vi "Equal.vi"(0 "VI Reference In":refnum<vi>, 1 "Label":string, 2 "delimiter (>>)":string=">>", 3 "Assert Only? (F)":bool, 5 "Control Name":string, 7 "Control Value":variant, 11 "Error In":errorcluster, 12 "Assert Interval(10 ms)":u32=10, 13 "Timeout(5 sec)":dbl=5.0) -> (4 "VI Reference Out":refnum<vi>, 15 "Error Out":errorcluster)   [LabVIEW 2016, in "AssertControlValueCompare.lvlib"]
doc: "Asserts if the numeric values of controls are almost equal.\n\nThe input control name is given as a string , incase of path, use delimiters inbetween the path.\nThis VI gets the value of the control, untill the value is almost equal to the input value."
uses:
  AssertControlValueCompare.lvlib
  Setup/GetControlRef/GetControlRefByPath.vi
  <vilib>/addons/_JKI Toolkits/Caraya/classes/Assert/Assert Equal Value and Type_Variant.vi
  <vilib>/addons/_JKI Toolkits/Caraya/classes/Assert/Assert.lvclass
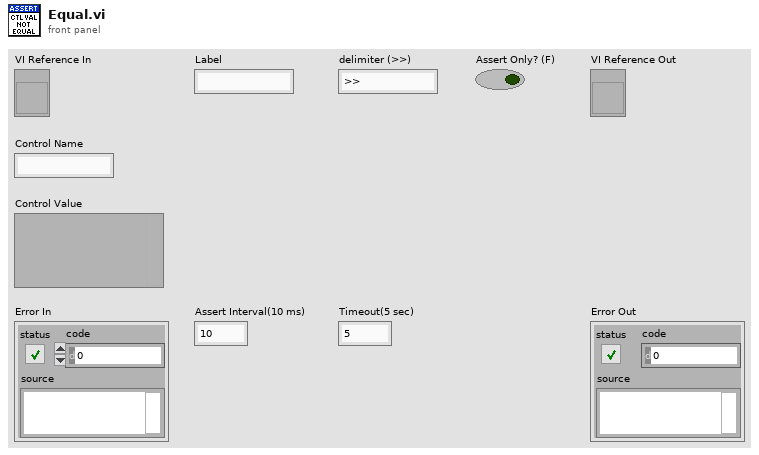
[diagram p1: front panel]
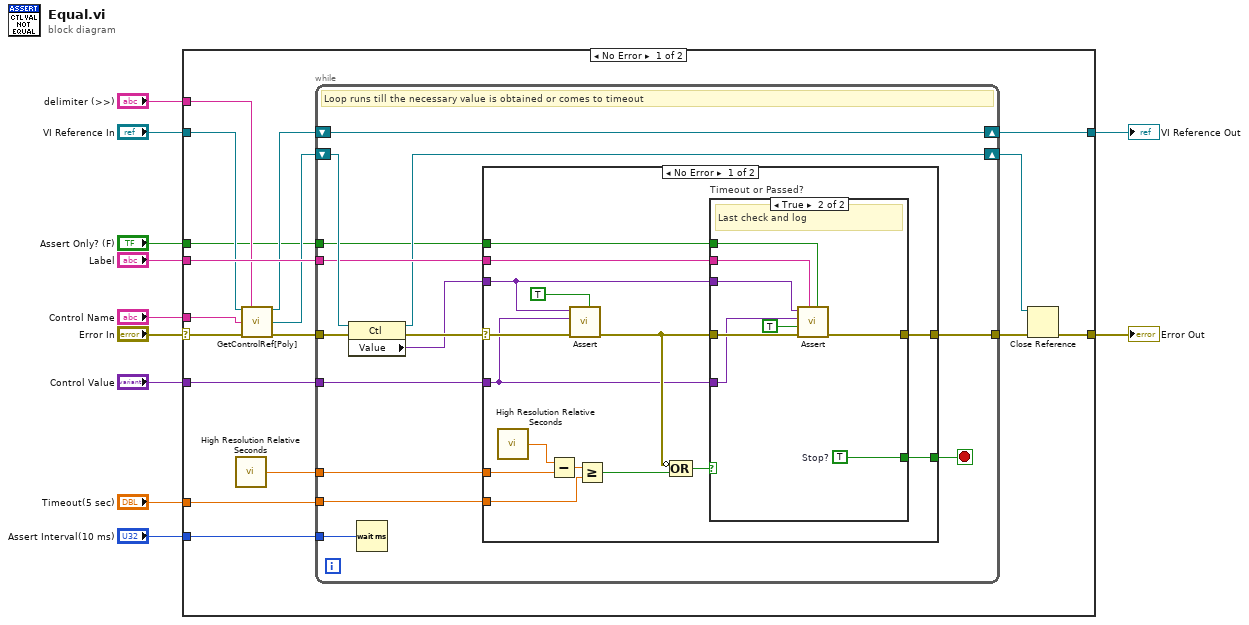
[diagram p0: block diagram]
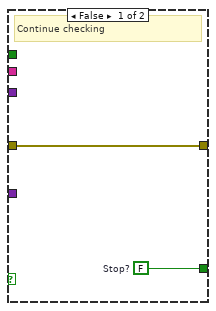
[diagram p2: hidden frame]
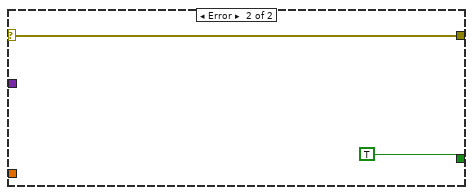
[diagram p3: hidden frame]
diagram:
  n1 = case shown="No Error" "Error In" {
    selector: "Error In" -> [w22 w71]
    tunnel: "Timeout(5 sec)" -> [w28 _]
    tunnel: [w27 w70] -> w10
    tunnel: "Control Value" -> [w26 _]
    tunnel: [w15 w71] -> w8
    tunnel: "Assert Interval(10 ms)" -> [w24 _]
    tunnel: "Label" -> [w23 _]
    tunnel: "VI Reference In" -> [w21 w70]
    tunnel: "Control Name" -> [w20 _]
    tunnel: "delimiter (>>)" -> [w13 _]
    tunnel: "Assert Only? (F)" -> [w12 _]
    frame No Error {
      n2 = call <vilib>:"High Resolution Relative Seconds.vi"() -> ("relative seconds"=w19:dbl)
      n3 = call-poly "GetControlRef[Poly].vi"("VI Reference In"=w21, "delimiter (>>)"=w13, "Control Path"=w20, "error In"=w22) -> ("VI Reference Out"=w17:refnum<vi>, "Ctl Refnum"=w16:refnum<vi>, "error out"=w18:errorcluster)  [unwired: 9 in]
      n4 = while {
        tunnel: w26 -> [w36]
        tunnel: w28 -> [w41]
        tunnel: w19 -> [w42]
        tunnel: w18 -> [w35]
        tunnel: [w39] -> w25
        tunnel: w24 -> [w37]
        tunnel: w23 -> [w31]
        shift-right: [w33] -> w27
        shift-left: w17 -> [w33]
        shift-right: [w30] -> w14
        shift-left: w16 -> [w34]
        tunnel: w12 -> [w29]
        stop <- w40 stop-if-true
        # "Loop runs till the necessary value is obtained or comes to timeout"
        n5 = property on="Property Node" class="Ctl"(reference=w34, error in=w35) -> (reference out=w30:refnum<vi>, error out=w38:errorcluster, "Value"=w32:variant)
        n6 = Wait (ms)(milliseconds to wait=w37) -> ()  [unwired: 1 out]
        n7 = case shown="No Error" w38 {
          selector: w38 -> [w53 w69]
          tunnel: w42 -> [w57 _]
          tunnel: w41 -> [w54 _]
          tunnel: [w44 TRUE] -> w40
          tunnel: [w45 w69] -> w39
          tunnel: w36 -> [w46 _]
          tunnel: w32 -> [w47 _]
          tunnel: w31 -> [w52 _]
          tunnel: w29 -> [w43 _]
          frame No Error {
            n8 = call <vilib>:"High Resolution Relative Seconds.vi"() -> ("relative seconds"=w56:dbl)
            n9 = Subtract(x=w56, y=w57) -> (x-y=w55:dbl)
            n10 = call-poly <vilib>:"Assert.vi"("Assert Only? (F)"=TRUE, "error in (no error)"=w53, "Y"=w46, "X"=w47) -> ("error out"=w50:errorcluster)  [unwired: 7 in]
            n11 = Greater Or Equal?(x=w55, y=w54) -> (x >= y?=w51:bool)
            n12 = Compound Arithmetic op=OR(invert w50, w51) -> (w49:bool)
            n13 = case "Timeout or Passed?" shown="True" w49 {
              tunnel: w50 -> [w59 w67]
              tunnel: w46 -> [_ w64]
              tunnel: w47 -> [_ w65]
              tunnel: w52 -> [_ w66]
              tunnel: [w59 w63] -> w45
              tunnel: [w58 w62] -> w44
              tunnel: w43 -> [_ w60]
              frame False {
                w58 = FALSE  # Stop?
                # "Continue checking"
              }
              frame True {
                w62 = TRUE  # Stop?
                # "Last check and log"
                n14 = call-poly <vilib>:"Assert.vi"("Assert Only? (F)"=w60, "Label"=w66, "error in (no error)"=w67, "Register with caller test (F)"=TRUE, "Y"=w64, "X"=w65) -> ("error out"=w63:errorcluster)  [unwired: 5 in]
              }
            }
          }
          frame Error {
          }
        }
      }
      n15 = Close Reference(reference=w14, error in (no error)=w25) -> (error out=w15:errorcluster)
    }
    frame Error {
    }
  }
  "Error Out" <- w8
  "VI Reference Out" <- w10
